vi "SR1.Reset.vi"(0 "i ref in":refnum<vi>, 5 "error in (no error)":errorcluster) -> (14 "i ref out":refnum<vi>, 19 "error out":errorcluster)   [LabVIEW 2014, in "SR1.lvlib"]
doc: "This is a Method that should be by changed by each daughter to class to implement a proper reset function."
uses:
  SR1.lvlib
  CS_Core/CSApplicationBaseClasses/DeviceBase/DeviceBase.lvlib
  CS_Core/CSApplicationBaseClasses/NABase/NABase.lvlib
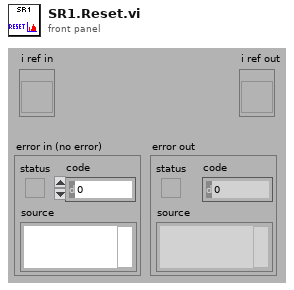
[diagram p1: front panel]
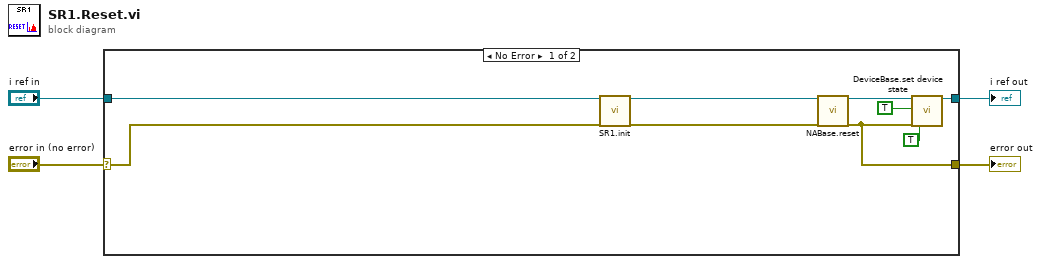
[diagram p0: block diagram]
diagram:
  n1 = case shown="No Error" "error in (no error)" {
    selector: "error in (no error)" -> [w8 w14]
    tunnel: "i ref in" -> [w7 w15]
    tunnel: [w9 w14] -> w3
    tunnel: [w13 w15] -> w2
    frame No Error {
      n2 = call "SR1.init.vi"("i ref in"=w7, "error in (no error)"=w8) -> ("i ref out"=w6:refnum<vi>, "error out"=w5:errorcluster)  [unwired: 16 in]
      n3 = call "NABase.reset.vi"("i ref in"=w6, "error in (no error)"=w5) -> ("i ref out"=w10:refnum<vi>, "error out"=w9:errorcluster)  [unwired: 16 in]
      n4 = call "DeviceBase.set device state.vi"("i ref in"=w10, "implicit"=TRUE, "error in (no error)"=w9, "mayResetError (FALSE)"=TRUE) -> ("i ref out"=w13:refnum<vi>)  [unwired: 13 in, 2 out]
    }
    frame Error {
    }
  }
  "error out" <- w3
  "i ref out" <- w2
